vi "Get Scale.vi"(5 "Read calibration":bool, 6 "Signal bits":i32=14, 7 "Number of stages":i32=6, 8 "error in (no error)":errorcluster, 9 "Range":dbl=1.0 format="%#_6eV", 10 "Channel":i32, 11 "RP Instrument in":refnum<class "RP Instrument.lvclass">) -> (0 "error out":errorcluster, 1 "slope":dbl, 2 "y intersept":dbl, 3 "RP Instrument out":refnum<class "RP Instrument.lvclass">, 4 "RP Calibration":T1)   [LabVIEW 2024, in "RP Instrument.lvclass"]
uses:
  RP Instrument.lvclass
  RP Calibration.ctl
  RP Calibration 4ch.ctl
  RP Channel Calibration.ctl
  RP Filter 4ch.ctl
  RP Channel Filter.ctl
  RP Calibration 2ch.ctl
  RP Instrument.lvclass/RP Instrument.ctl
  Read Decimation.vi
  RP Communicator/RP Communicator.lvclass
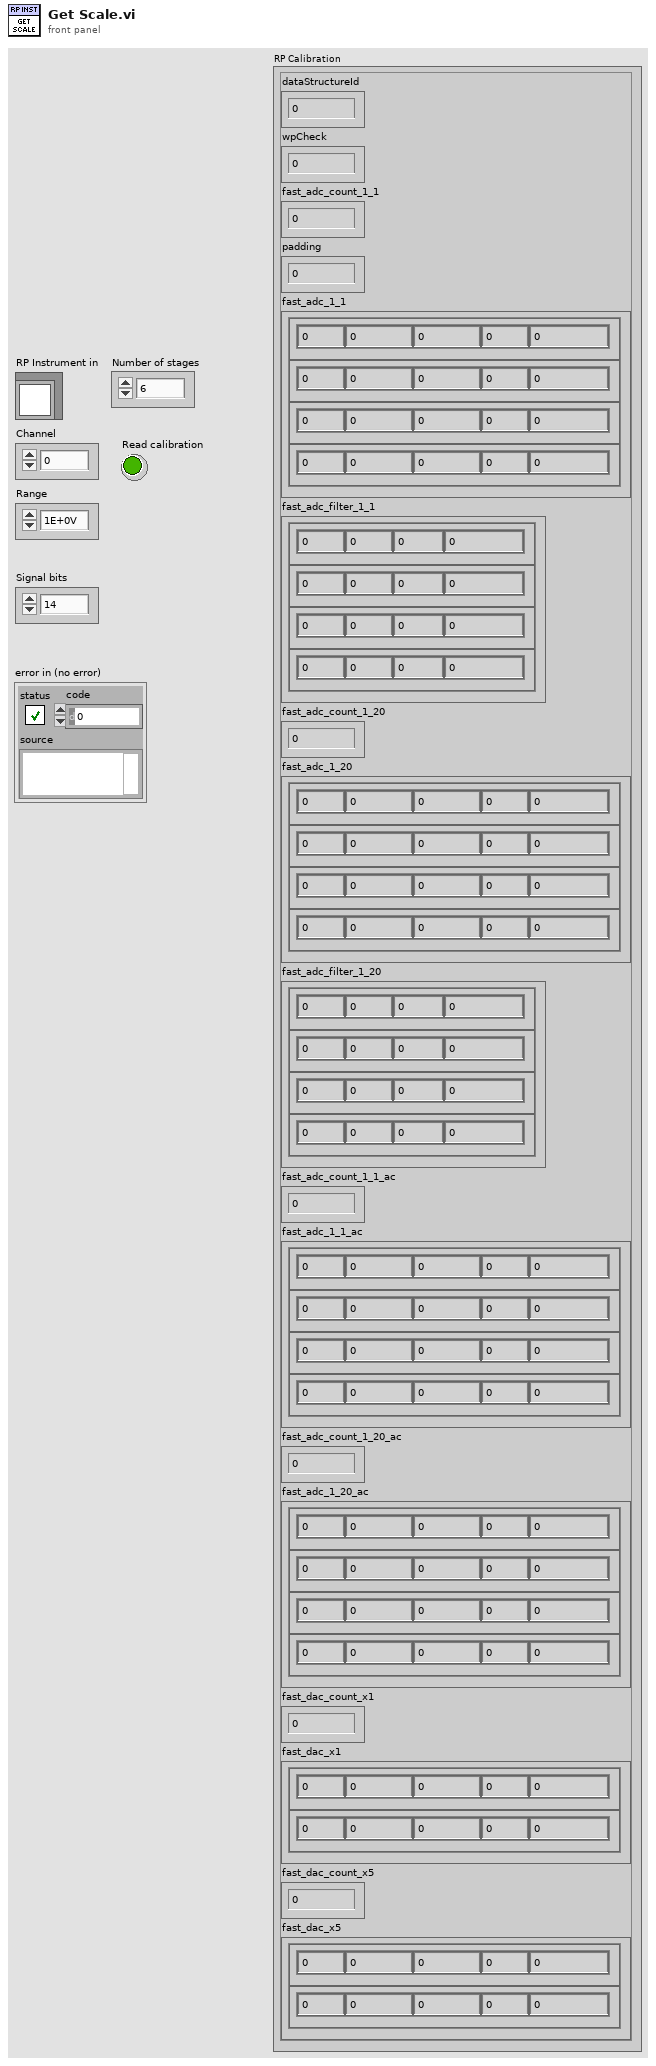
[diagram p1: front panel]
types:
  T1 = typedef "RP Calibration.ctl" = cluster{"dataStructureId":u8, "wpCheck":u8, "fast_adc_count_1_1":u16, "padding":u32, "fast_adc_1_1":T2, "fast_adc_filter_1_1":T4, "fast_adc_count_1_20":u64, "fast_adc_1_20":T2, "fast_adc_filter_1_20":T4, "fast_adc_count_1_1_ac":u64, "fast_adc_1_1_ac":T2, "fast_adc_count_1_20_ac":u64, "fast_adc_1_20_ac":T2, "fast_dac_count_x1":u64, "fast_dac_x1":T6, "fast_dac_count_x5":u64, "fast_dac_x5":T6}
  T2 = typedef "RP Calibration 4ch.ctl" = cluster{"ch_0":T3, "ch_1":T3, "ch_2":T3, "ch_3":T3}
  T3 = typedef "RP Channel Calibration.ctl" = cluster{"baseScale":sgl, "calibValue":u32, "offset":i32, "padding 2":i32, "gainCalc":dbl}
  T4 = typedef "RP Filter 4ch.ctl" = cluster{"ch_0":T5, "ch_1":T5, "ch_2":T5, "ch_3":T5}
  T5 = typedef "RP Channel Filter.ctl" = cluster{"aa":u32, "bb":u32, "pp":u32, "kk":u32}
  T6 = typedef "RP Calibration 2ch.ctl" = cluster{"ch_0":T3, "ch_1":T3}
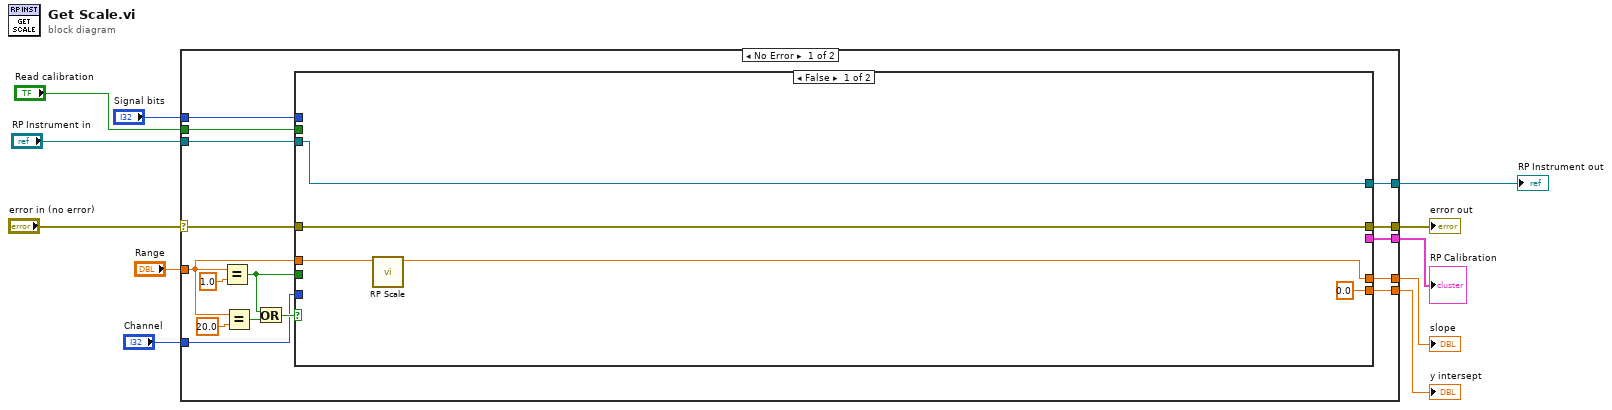
[diagram p0: block diagram]
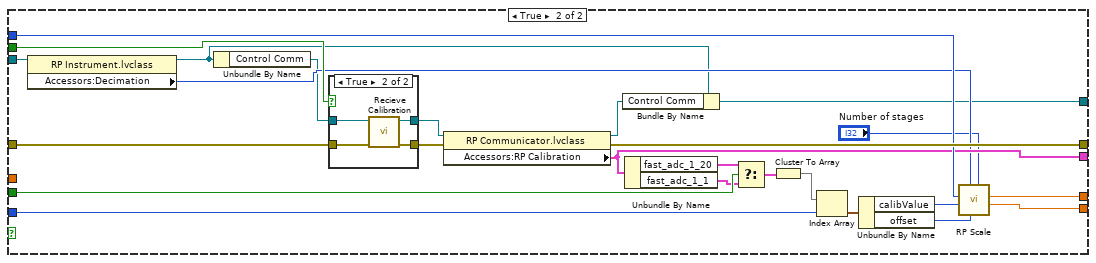
[diagram p2: hidden frame]
diagram:
  n1 = case shown="No Error" "error in (no error)" {
    selector: "error in (no error)" -> [w18 w65]
    tunnel: [w17 w65] -> w10
    tunnel: [w12 w64] -> w8
    tunnel: "RP Instrument in" -> [w24 w64]
    tunnel: "Range" -> [w20 _]
    tunnel: "Channel" -> [w23 _]
    tunnel: [w21 _] -> w5
    tunnel: [w19 _] -> w4
    tunnel: "Signal bits" -> [w15 _]
    tunnel: [w14 _] -> w2
    tunnel: "Read calibration" -> [w13 _]
    frame No Error {
      n2 = Equal?(x=w20, y=1.0) -> (x = y?=w16:bool)
      n3 = Equal?(x=w20, y=20.0) -> (x = y?=w22:bool)
      n4 = Or(x=w16, y=w22) -> (x .or. y?=w25:bool)
      n5 = case shown="False" w25 {
        tunnel: w24 -> [w28 w55]
        tunnel: w23 -> [_ w57]
        tunnel: w16 -> [_ w56]
        tunnel: [0.0 w52] -> w21
        tunnel: w20 -> [w31 _]
        tunnel: [w30 w53] -> w19
        tunnel: w18 -> [w29 w49]
        tunnel: [w29 w54] -> w17
        tunnel: w15 -> [_ w51]
        tunnel: [_ w50] -> w14
        tunnel: w13 -> [_ w48]
        tunnel: [w28 w45] -> w12
        frame False {
          n6 = call "RP Scale.vi"("Range"=w31) -> ("Slope"=w30:dbl)  [unwired: 8 in, 2 out]
        }
        frame True {
          n7 = property class="RP Instrument.lvclass"(reference=w55) -> (reference out=w46:refnum<class "RP Instrument.lvclass">, "Accessors:Decimation"=w47:i32)  [unwired: 1 in, 1 out]
          n8 = Unbundle By Name(w46) -> ("Control Comm"=w42:refnum<class "RP Communicator.lvclass">)
          n9 = case shown="True" w48 {
            tunnel: w42 -> [w59 w63]
            tunnel: [w59 w62] -> w41
            tunnel: w49 -> [w58 w61]
            tunnel: [w58 w60] -> w40
            frame False {
            }
            frame True {
              n10 = call-dynamic "Recieve Calibration.vi"("error in (no error)"=w61, "RP Communicator in"=w63) -> ("error out"=w60:errorcluster, "RP Communicator out"=w62:refnum<class "RP Communicator.lvclass">)  [unwired: 7 in, 1 out]
            }
          }
          n11 = property class="RP Communicator.lvclass"(reference=w41, error in=w40) -> (reference out=w44:refnum<class "RP Communicator.lvclass">, error out=w54:errorcluster, "Accessors:RP Calibration"=w50:T1)
          n12 = Bundle By Name(cluster=w46, "Control Comm"=w44) -> (w45:refnum<class "RP Instrument.lvclass">)
          n13 = Unbundle By Name(w50) -> ("fast_adc_1_20"=w39:T2, "fast_adc_1_1"=w38:T2)
          n14 = Select(t=w39, s=w56, f=w38) -> (s? t:f=w37:T2)
          n15 = Cluster To Array(cluster=w37) -> (array=w36:T3[])
          n16 = Index Array(array=w36, index=w57) -> (element=w35:T3)
          n17 = Unbundle By Name(w35) -> ("calibValue"=w33:u32, "offset"=w34:i32)
          n18 = call "RP Scale.vi"("Number of stages"="Number of stages", "EEPROM offset"=w34, "Decimation"=w47, "EEPROM range"=w33, "Signal bits"=w51) -> ("y intersept"=w52:dbl, "Calibrated slope"=w53:dbl)  [unwired: 4 in, 1 out]
        }
      }
    }
    frame Error {
    }
  }
  "error out" <- w10
  "RP Instrument out" <- w8
  "slope" <- w4
  "y intersept" <- w5
  "RP Calibration" <- w2
